vi "motor.vi"() -> ()   [LabVIEW 2013]
panel:
  in  "Start":bool
  in  "?":bool
  in  "Step Size (nm)":dbl(slide) scale=0.0..1000.0
  in  "?":bool
  in  "Frequency (Hz)":dbl(knob) scale=1.0..500.0 scale format="%#_3f"
  # "DCP"
  # "PUMP"
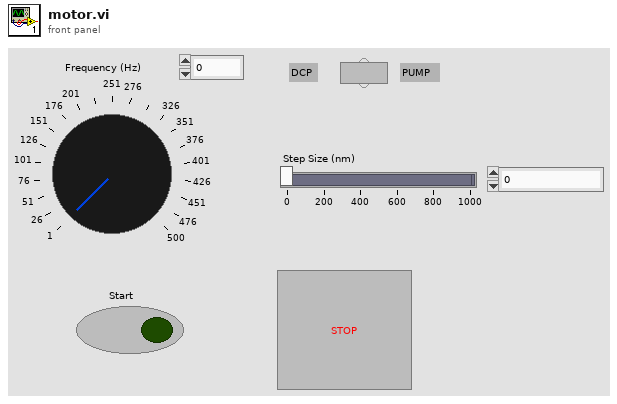
[diagram p1: front panel]
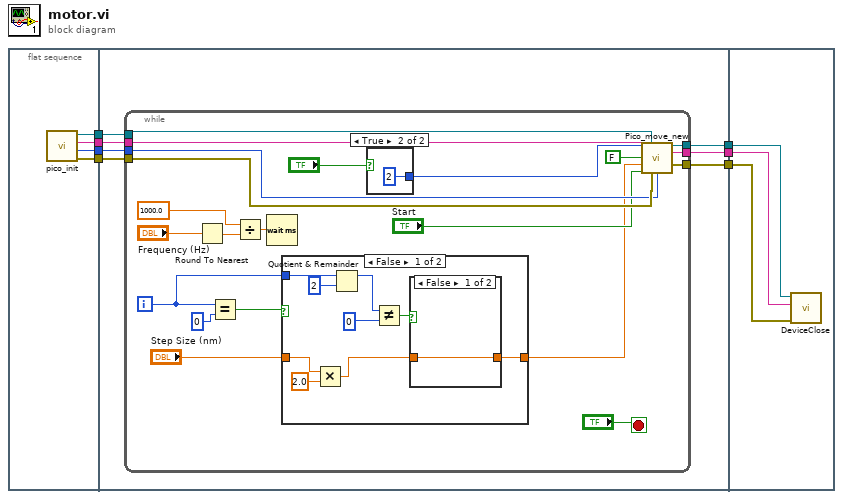
[diagram p0: block diagram]
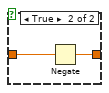
[diagram p2: hidden frame]
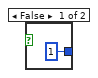
[diagram p4: hidden frame]
diagram:
  n1 = flat-sequence {
    tunnel: [w11] -> w7
    tunnel: [w10] -> w6
    tunnel: [w9] -> w5
    tunnel: [w8] -> w4
    tunnel: w7 -> [w18]
    tunnel: w6 -> [w17]
    tunnel: w5 -> [w16]
    tunnel: w4 -> [w15]
    tunnel: [w14] -> w3
    tunnel: [w13] -> w2
    tunnel: [w12] -> w1
    tunnel: w3 -> [w57]
    tunnel: w2 -> [w56]
    tunnel: w1 -> [w55]
    frame #0 {
      n2 = call "pico_init.vi"() -> ("error out 3"=w8:errorcluster, "ID"=w9:i32, "key"=w10:string, "CmdLib Out"=w11:refnum<k24>)  [unwired: 8 in]
    }
    frame #1 {
      n3 = while {
        tunnel: w18 -> [w39]
        tunnel: w17 -> [w38]
        tunnel: w16 -> [w35]
        tunnel: w15 -> [w37]
        tunnel: [w26] -> w14
        tunnel: [w25] -> w13
        tunnel: [w24] -> w12
        i -> [w19]
        stop <- "?" stop-if-true
        n4 = Round To Nearest(number="Frequency (Hz)") -> (nearest integer value=w21:dbl)
        n5 = Equal?(x=w19, y=0) -> (x = y?=w30:bool)
        n6 = Divide(x=1000.0 ("y"), y=w21) -> (x/y=w22:dbl)
        n7 = Wait (ms)(milliseconds to wait=w22) -> ()  [unwired: 1 out]
        n8 = case shown="False" w30 {
          tunnel: "Step Size (nm)" -> [w40 w52]
          tunnel: [w45 w52] -> w28
          tunnel: w19 -> [w41 _]
          frame False {
            n9 = Multiply(x=w40, y=2.0) -> (x*y=w43:dbl)
            n10 = Quotient & Remainder(x=w41, y=2) -> (x-y*floor(x/y)=w47:i32)  [unwired: 1 out]
            n11 = Not Equal?(x=w47, y=0) -> (x != y?=w48:bool)
            n12 = case shown="False" w48 {
              tunnel: [w49 w51] -> w45
              tunnel: w43 -> [w49 w50]
              frame False {
              }
              frame True {
                n13 = Negate(x=w50) -> (-x=w51:dbl)
              }
            }
          }
          frame True {
          }
        }
        n14 = case shown="True" "?" {
          tunnel: [1 ("Motor") 2 ("Motor")] -> w34
          frame False {
          }
          frame True {
          }
        }
        n15 = call "Pico_move_new.vi"("Motor"=w34, "CmdLib Out"=w39, "DeviceKey Out"=w38, "Boolean 2"=FALSE, "Relative Steps"=w28, "Boolean"="Start", "error out"=w37, "Device Address Out"=w35) -> ("CmdLib Out"=w26:refnum<k24>, "DeviceKey Out"=w25:string, "error out 2"=w24:errorcluster)  [unwired: 4 in, 1 out]
      }
    }
    frame #2 {
      n16 = call <instrlib>:"DeviceClose.vi"("error in (no error)"=w55, "DeviceKey In"=w56, "CmdLib In"=w57) -> ()  [unwired: 2 in, 3 out]
    }
  }
